vi "armSetpoints.vi"() -> ()   [LabVIEW 2020]
panel:
  in  "Spool pos":dbl
  in  "Arm pos":dbl
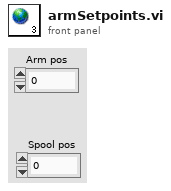
[diagram p1: front panel]
diagram:
